vi "Set Limits.vi"(8 "error in":errorcluster, 11 "Keithley 2400 in":refnum<class "Keithley 2400.lvclass">) -> (0 "error out":errorcluster, 3 "Keithley 2400 out":refnum<class "Keithley 2400.lvclass">)   [LabVIEW 2011, in "Keithley 2400.lvclass"]
uses:
  Keithley 2400.lvclass
  Keithley 2400.lvclass/Keithley 2400.ctl
  <instrlib>/Keithley 24XX/Keithley 24XX.lvlib
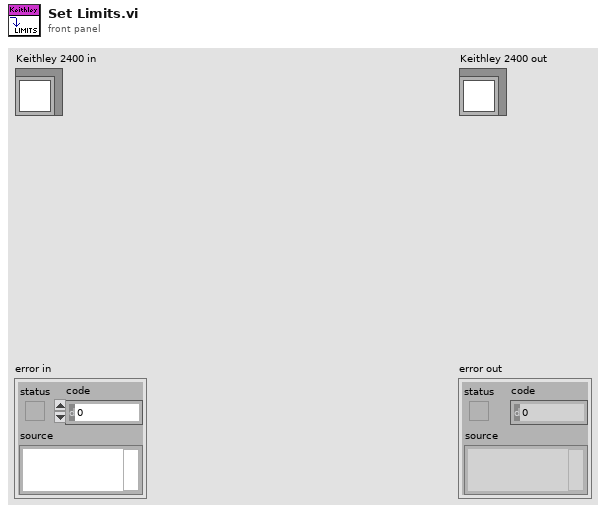
[diagram p1: front panel]
types:
  T1 = typedef "Power Supply.lvclass/Source Mode.ctl" = enum16{"Volts", "Current"}
  T2 = typedef "Power Supply.lvclass/Protection Limits.ctl" = cluster{"Voltage Limit":dbl, "Voltage Limit Units":T3, "Current Limit":dbl, "Current Limit Units":T4, "Voltage Trip/Cmpl":dbl, "Voltage Trip/Cmpl Units":T3, "Current Trip/Cmpl":dbl, "Current Trip/Cmpl Units":T4}
  T3 = typedef "Power Supply.lvclass/Voltage Units.ctl" = enum16{"volts", "millivolts", "microvolts"}
  T4 = typedef "Power Supply.lvclass/Current Units.ctl" = enum16{"amps", "milliamps", "microamps", "nanoamps"}
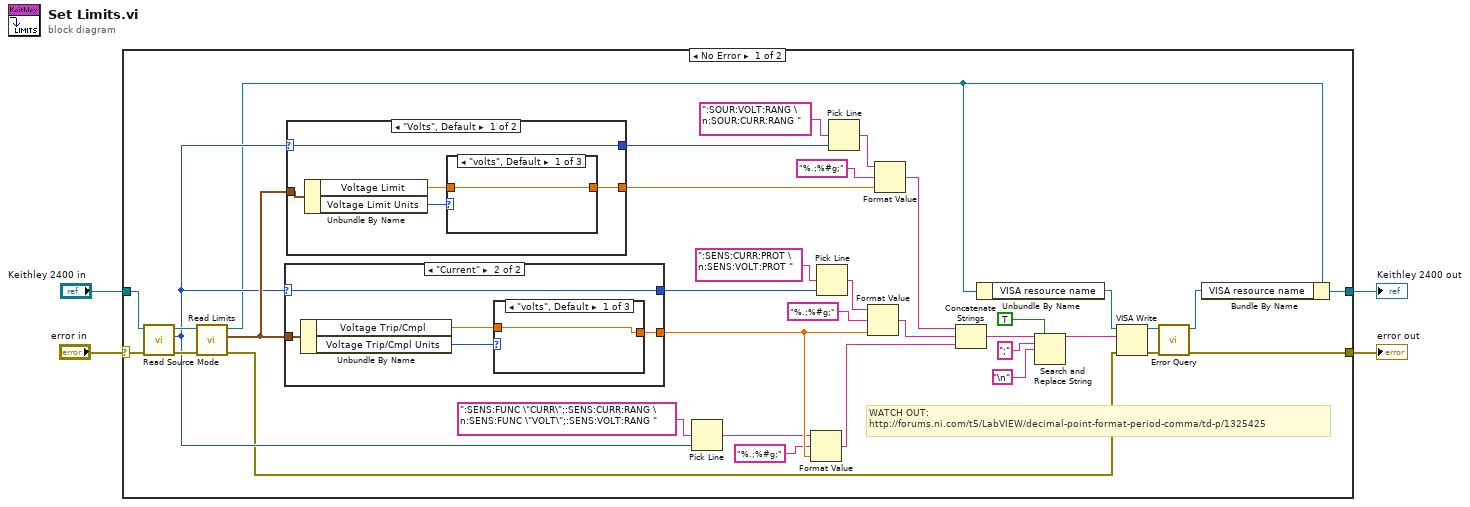
[diagram p0: block diagram]
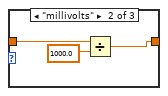
[diagram p2: hidden frame]
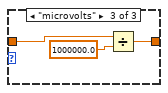
[diagram p3: hidden frame]
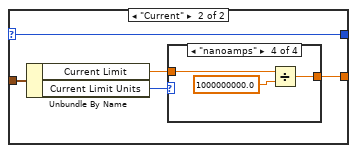
[diagram p4: hidden frame]
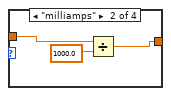
[diagram p6: hidden frame]
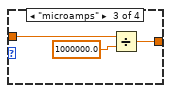
[diagram p7: hidden frame]
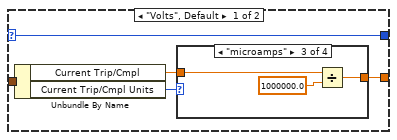
[diagram p8: hidden frame]
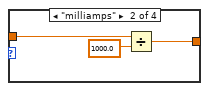
[diagram p10: hidden frame]
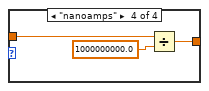
[diagram p11: hidden frame]
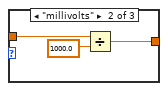
[diagram p12: hidden frame]
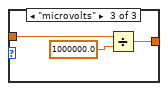
[diagram p13: hidden frame]
diagram:
  n1 = case shown="No Error" "error in" {
    selector: "error in" -> [w37 w95]
    tunnel: [w22 w95] -> w3
    tunnel: [w32 w94] -> w1
    tunnel: "Keithley 2400 in" -> [w39 w94]
    frame No Error {
      # "WATCH OUT:\nhttp://forums.ni.com/t5/LabVIEW/decimal-point-format-period-comma/td-p/1325425"
      n2 = call-dynamic "Read Source Mode.vi"("error in (no error)"=w37, "Power Supply in"=w39) -> ("error out"=w36:errorcluster, "Source Mode"=w29:T1, "Power Supply out"=w38:refnum<class "Keithley 2400.lvclass">)  [unwired: 7 in]
      n3 = call-dynamic "Read Limits.vi"("error in (no error)"=w36, "Power Supply in"=w38) -> ("error out"=w16:errorcluster, "Protection Limits"=w30:T2, "Power Supply out"=w8:refnum<class "Keithley 2400.lvclass">)  [unwired: 7 in]
      n4 = case shown="\"Current\"" w29 {
        selector: w29 -> [w67 w82]
        tunnel: w30 -> [w71 w86]
        tunnel: [w68 w83] -> w31
        tunnel: [w67 w82] -> w6
        frame "Volts", Default {
          n5 = Unbundle By Name(w71) -> ("Current Trip/Cmpl"=w69:dbl, "Current Trip/Cmpl Units"=w70:T4)
          n6 = case shown="\"microamps\"" w70 {
            tunnel: w69 -> [w72 w75 w78 w81]
            tunnel: [w72 w74 w76 w79] -> w68
            frame "amps", Default {
            }
            frame "milliamps" {
              n7 = Divide(x=w75, y=1000.0) -> (x/y=w74:dbl)
            }
            frame "microamps" {
              n8 = Divide(x=w78, y=1000000.0) -> (x/y=w76:dbl)
            }
            frame "nanoamps" {
              n9 = Divide(x=w81, y=1000000000.0) -> (x/y=w79:dbl)
            }
          }
        }
        frame "Current" {
          n10 = Unbundle By Name(w86) -> ("Voltage Trip/Cmpl"=w84:dbl, "Voltage Trip/Cmpl Units"=w85:T3)
          n11 = case shown="\"volts\", Default" w85 {
            tunnel: w84 -> [w87 w90 w93]
            tunnel: [w87 w88 w91] -> w83
            frame "volts", Default {
            }
            frame "millivolts" {
              n12 = Divide(x=w90, y=1000.0) -> (x/y=w88:dbl)
            }
            frame "microvolts" {
              n13 = Divide(x=w93, y=1000000.0) -> (x/y=w91:dbl)
            }
          }
        }
      }
      n14 = case shown="\"Volts\", Default" w29 {
        selector: w29 -> [w40 w52]
        tunnel: w30 -> [w44 w56]
        tunnel: [w41 w53] -> w26
        tunnel: [w40 w52] -> w7
        frame "Volts", Default {
          n15 = Unbundle By Name(w44) -> ("Voltage Limit"=w42:dbl, "Voltage Limit Units"=w43:T3)
          n16 = case shown="\"volts\", Default" w43 {
            tunnel: w42 -> [w45 w48 w51]
            tunnel: [w45 w47 w49] -> w41
            frame "volts", Default {
            }
            frame "millivolts" {
              n17 = Divide(x=w48, y=1000.0) -> (x/y=w47:dbl)
            }
            frame "microvolts" {
              n18 = Divide(x=w51, y=1000000.0) -> (x/y=w49:dbl)
            }
          }
        }
        frame "Current" {
          n19 = Unbundle By Name(w56) -> ("Current Limit"=w54:dbl, "Current Limit Units"=w55:T4)
          n20 = case shown="\"nanoamps\"" w55 {
            tunnel: w54 -> [w57 w60 w63 w65]
            tunnel: [w57 w58 w61 w64] -> w53
            frame "amps", Default {
            }
            frame "milliamps" {
              n21 = Divide(x=w60, y=1000.0) -> (x/y=w58:dbl)
            }
            frame "microamps" {
              n22 = Divide(x=w63, y=1000000.0) -> (x/y=w61:dbl)
            }
            frame "nanoamps" {
              n23 = Divide(x=w65, y=1000000000.0) -> (x/y=w64:dbl)
            }
          }
        }
      }
      n24 = Pick Line(multi-line string=":SENS:FUNC \"CURR\";:SENS:CURR:RANG \n:SENS:FUNC \"VOLT\";:SENS:VOLT:RANG ", line index=w29) -> (output string=w20:string)  [unwired: 1 in]
      n25 = Format Value(string ("")=w20, format string="%.;%#g;", value (0)=w31) -> (output string=w13:string)
      n26 = Pick Line(multi-line string=":SENS:CURR:PROT \n:SENS:VOLT:PROT ", line index=w6) -> (output string=w34:string)  [unwired: 1 in]
      n27 = Pick Line(multi-line string=":SOUR:VOLT:RANG \n:SOUR:CURR:RANG ", line index=w7) -> (output string=w28:string)  [unwired: 1 in]
      n28 = Format Value(string ("")=w34, format string="%.;%#g;", value (0)=w31) -> (output string=w14:string)
      n29 = Format Value(string ("")=w28, format string="%.;%#g;", value (0)=w26) -> (output string=w15:string)
      n30 = Concatenate Strings(w15, w14, w13) -> (w9:string)
      n31 = Unbundle By Name(w8) -> ("VISA resource name"=w17:refnum<visa-resource-name>)
      n32 = Search and Replace String(replace all?=TRUE ("replace all? (F)"), input string=w9, search string=";", replace string="\n") -> (result string=w5:string)  [unwired: 4 in, 3 out]
      n33 = VISA Write(VISA resource name=w17, write buffer=w5, error in (no error)=w16) -> (VISA resource name out=w24:refnum<visa-resource-name>, error out=w23:errorcluster)  [unwired: 1 out]
      n34 = call <instrlib>:"Error Query.vi"("error in (no error)"=w23, "VISA resource name"=w24) -> ("error out"=w22:errorcluster, "VISA resource name out"=w21:refnum<visa-resource-name>)  [unwired: 6 in, 2 out]
      n35 = Bundle By Name(cluster=w8, "VISA resource name"=w21) -> (w32:refnum<class "Keithley 2400.lvclass">)
    }
    frame Error {
    }
  }
  "error out" <- w3
  "Keithley 2400 out" <- w1
